vi "test Update Device.vi"() -> ()   [LabVIEW 2019]
uses:
  <vilib>/Utility/config.llb/Read Key (String).vi
  <vilib>/Utility/config.llb/NI_LVConfig.lvlib
panel:
  out "Array":T1(array[cluster])
  out "error out":errorcluster
  in  "configuration file path":path
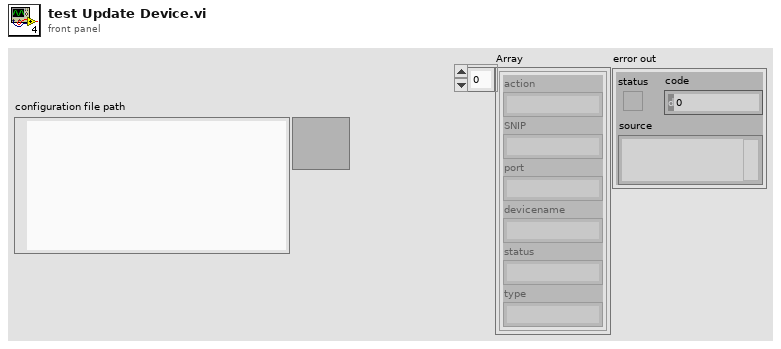
[diagram p1: front panel]
types:
  T1 = cluster{"action":string, "SNIP":string, "port":string, "devicename":string, "status":string, "type":string}[]
  T2 = typedef "NI_LVConfig.lvlib/Config Data RefNum.ctl" = refnum<k1>
  T3 = cluster{"action":string, "SNIP":string, "port":string, "devicename":string, "status":string, "type":string}
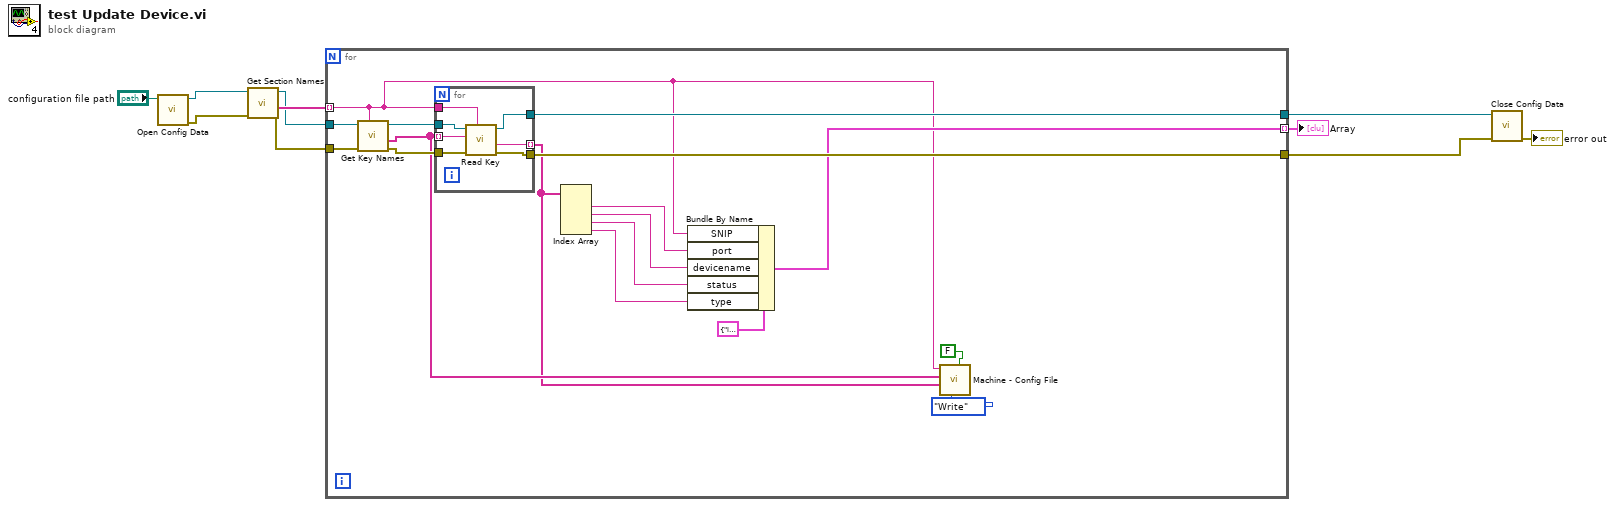
[diagram p0: block diagram]
diagram:
  n1 = call <vilib>:"Open Config Data.vi"("configuration file path"="configuration file path") -> ("error out"=w9:errorcluster, "refnum"=w10:T2)  [unwired: 8 in, 1 out]
  n2 = call <vilib>:"Get Section Names.vi"("error in (no error)"=w9, "refnum"=w10) -> ("error out"=w4:errorcluster, "section names"=w8:string[], "refnum out"=w7:T2)  [unwired: 7 in]
  n3 = for {
    tunnel: w8 -> [w13] mode=indexing
    tunnel: [w16] -> w1 mode=indexing
    tunnel: w7 -> [w27]
    tunnel: [w25] -> w6
    tunnel: w4 -> [w24]
    tunnel: [w22] -> w3
    n4 = call <vilib>:"Get Key Names.vi"("section"=w13, "error in (no error)"=w24, "refnum"=w27) -> ("error out"=w23:errorcluster, "key names"=w12:string[], "refnum out"=w26:T2)  [unwired: 5 in, 1 out]
    n5 = for {
      tunnel: w12 -> [w34] mode=indexing
      tunnel: w13 -> [w33]
      tunnel: [w32] -> w11 mode=indexing
      tunnel: w26 -> [w31]
      tunnel: [w30] -> w25
      tunnel: w23 -> [w29]
      tunnel: [w28] -> w22
      n6 = call-poly <vilib>:"Read Key.vi"("section"=w33, "error in (no error)"=w29, "key"=w34, "refnum"=w31) -> ("error out"=w28:errorcluster, "value"=w32:string, "refnum out"=w30:T2)  [unwired: 4 in, 1 out]
    }
    n7 = Index Array(array=w11) -> (element #1=w20:string, element #2=w19:string, element #3=w18:string, element #4=w17:string)  [unwired: 4 in]
    n8 = Bundle By Name(cluster=T3 {"action"="insert", "SNIP"="192.168.1.7", "port"="4007", "devicename"="test3", "status"="1", "type"="flowtron"}, "SNIP"=w13, "port"=w20, "devicename"=w19, "status"=w18, "type"=w17) -> (w16:T3)
    n9 = call "Machine - Config File.vi"("Setting"=FALSE, "Action"=enum16{"Write", "Read", "Read All", "Remove"}."Write", "Value"=w11, "Key Name"=w12, "IP/SN"=w13) -> ()  [unwired: 5 in, 2 out]
  }
  "Array" <- w1
  n10 = call <vilib>:"Close Config Data.vi"("error in (no error)"=w3, "refnum"=w6) -> ("error out"=→"error out":errorcluster)  [unwired: 8 in, 1 out]
